vi "Default Instrument Setup.vi"(8 "error in (no error)":errorcluster, 11 "VISA resource name":refnum<visa-resource-name>) -> (0 "error out":errorcluster, 3 "VISA resource name out":refnum<visa-resource-name>)   [LabVIEW 2011, in "Template - Register.lvlib"]
doc: "This Utility VI sends a default command string to the instrument whenever a new VISA session is opened, or the instrument is reset. Use this VI as a subVI for the Initialize and Reset VIs. Altering this VI could cause these two VIs to operate incorrectly."
uses:
  <instrlib>/_Template - Register/Template - Register.lvlib
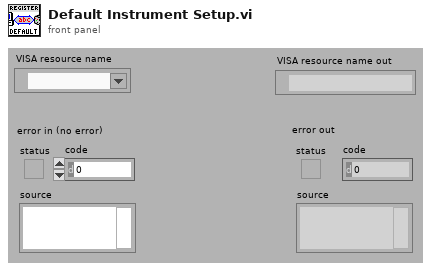
[diagram p1: front panel]
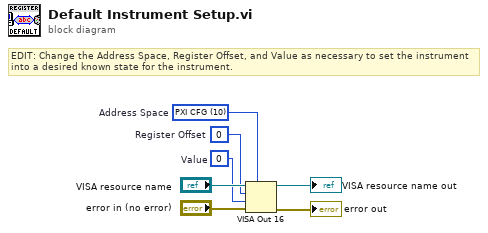
[diagram p0: block diagram]
diagram:
  w1 = u16 0  # Value
  w2 = u32 0  # Register Offset
  w3 = u16 10 items=["A16"=1, "A24"=2, "A32"=3, "PXI CFG"=10, "PXI BAR0"=11, "PXI BAR1"=12, "PXI BAR2"=13, "PXI BAR3"=14, "PXI BAR4"=15, "PXI BAR5"=16]  # Address Space
  # "EDIT: Change the Address Space, Register Offset, and Value as necessary to set the instrument\ninto a desired known state for the instrument."
  n1 = VISA Out 16(7:w3, 8:"error in (no error)", 9:w1, 10:w2, 11:"VISA resource name") -> (0:→"error out":errorcluster, 3:→"VISA resource name out":refnum<visa-resource-name>)
